vi "vapor_temp_psat_density.vi"(0 "Vapor Temp [C]":dbl[](array[numeric])) -> (1 "Psat Vapor":dbl[](array[numeric]), 3 "Vapor Density":dbl[](array[numeric]))   [LabVIEW 2017]
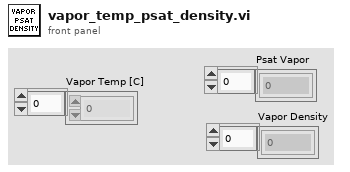
[diagram p1: front panel]
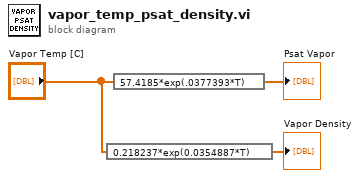
[diagram p0: block diagram]
diagram:
  n1 = expression code="0.218237*exp(0.0354887*T)"("Vapor Temp [C]") -> (→"Vapor Density":dbl[])
  n2 = expression code="57.4185*exp(.0377393*T)"("Vapor Temp [C]") -> (→"Psat Vapor":dbl[])
